vi "testing average temperatures.vi"() -> ()   [LabVIEW 2019]
panel:
  in  "Temp Scale":bool
  in  "stop":bool
  out "average":dbl
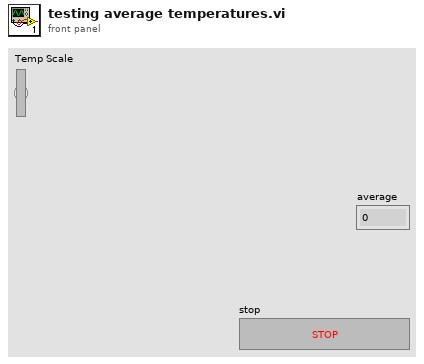
[diagram p1: front panel]
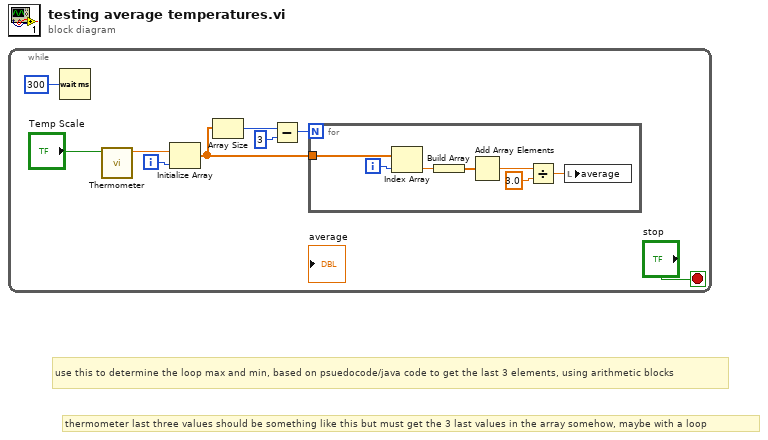
[diagram p0: block diagram]
diagram:
  # "use this to determine the loop max and min, based on psuedocode/java code to get the last 3 elements, using arithmetic blocks"
  # "thermometer last three values should be something like this but must get the 3 last values in the array somehow, maybe with a loop"
  n1 = while {
    i -> [w6]
    stop <- "stop" stop-if-true
    n2 = Wait (ms)(milliseconds to wait=u32 300) -> ()  [unwired: 1 out]
    n3 = call "Thermometer.vi"("Temp Scale"="Temp Scale") -> ("Temperature"=w7:dbl)  [unwired: 10 in]
    n4 = Initialize Array(w7, w6) -> (w2:dbl[])
    n5 = Array Size(array=w2) -> (size(s)=w5:i32)
    n6 = Subtract(x=w5, y=3) -> (x-y=w3:i32)
    n7 = for {
      N: w3 -> [_]
      tunnel: w2 -> [w16]
      i -> [w15]
      n8 = Index Array(array=w16, index=w15) -> (element=w14:dbl)
      n9 = Build Array(w14) -> (w13:dbl[])
      n10 = Add Array Elements(numeric array=w13) -> (sum=w12:dbl)
      n11 = Divide(x=w12, y=3.0) -> (x/y=w10:dbl)
      n12 = local write "average"(w10) -> ()
    }
  }
